vi "S2C_CMD_NumberCheck.vi"(8 "Error In":errorcluster, 11 "String In":string) -> (0 "Error Out":errorcluster, 2 "Is Number?":bool, 3 "String Out":string)   [LabVIEW 2024]
doc: "Checks if the input string is a number and removes any quotes if it is."
uses:
  <vilib>/Utility/error.llb/Trim Whitespace One-Sided.vi
  <vilib>/regexp/Match Regular Expression.xnode
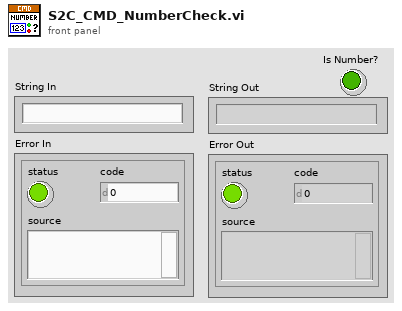
[diagram p1: front panel]
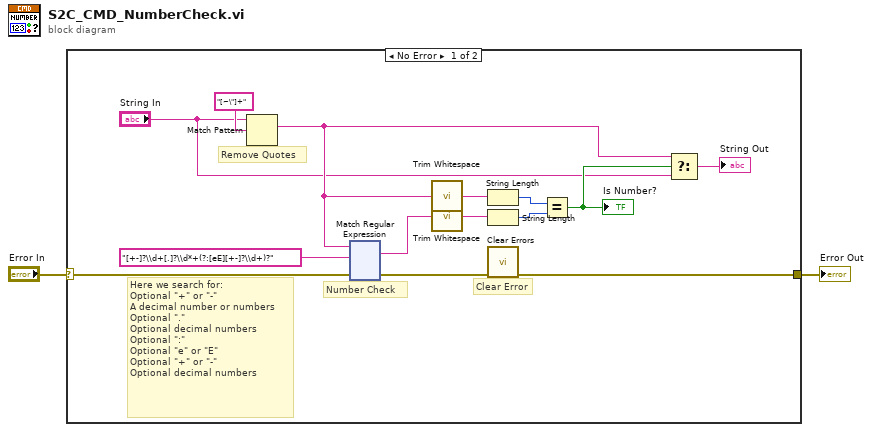
[diagram p0: block diagram]
diagram:
  n1 = case shown="No Error" "Error In" {
    selector: "Error In" -> [w13 w134]
    tunnel: [w10 w134] -> w1
    frame No Error {
      # "Remove Quotes"
      # "Clear Error"
      # "Number Check"
      # "Here we search for:\nOptional \"+\" or \"-\"\nA decimal number or numbers\nOptional \".\"\nOptional decimal numbers\nOptional \":\"\nOptional \"e\" or \"E\"\nOptional \"+\" or \"-\"\nOptional decimal numbers"
      n2 = Match Pattern(string="String In", regular expression="[~\"]+") -> (match substring=w6:string)  [unwired: 1 in, 3 out]
      n3 = xnode "Match Regular Expression"("input string"=w6, "regular expression"="[+-]?\\d+[.]?\\d*+(?:[eE][+-]?\\d+)?", "error in"=w13) -> ("whole match"=w11:string, "error out"=w12:errorcluster)  [unwired: 3 in, 3 out]
      n4 = call <vilib>:"Trim Whitespace.vi"("string"=w6) -> ("trimmed string"=w4:string)  [unwired: 1 in]
      n5 = call <vilib>:"Trim Whitespace.vi"("string"=w11) -> ("trimmed string"=w3:string)  [unwired: 1 in]
      n6 = String Length(string=w4) -> (length=w15:i32)
      n7 = String Length(string=w3) -> (length=w14:i32)
      n8 = call <vilib>:"Clear Errors.vi"("error in (no error)"=w12) -> ("error out"=w10:errorcluster)  [unwired: 5 in, 1 out]
      n9 = Equal?(x=w15, y=w14) -> (x = y?=w9:bool)
      "Is Number?" <- w9
      n10 = Select(t=w6, s=w9, f="String In") -> (s? t:f=→"String Out":string)
    }
    frame Error {
    }
  }
  "Error Out" <- w1
